vi "crh_xcopy.vi"() -> ()   [LabVIEW 2012]
panel:
  out "concatenated string":string
  out "OK 2":bool
  out "concatenated string 2":string
  out "folder 2":string
  out "OK":bool
  in  "folder":string="QAMT01\\CRH3605"
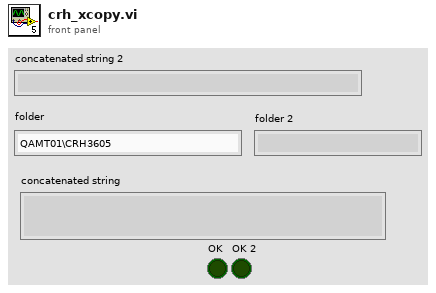
[diagram p1: front panel]
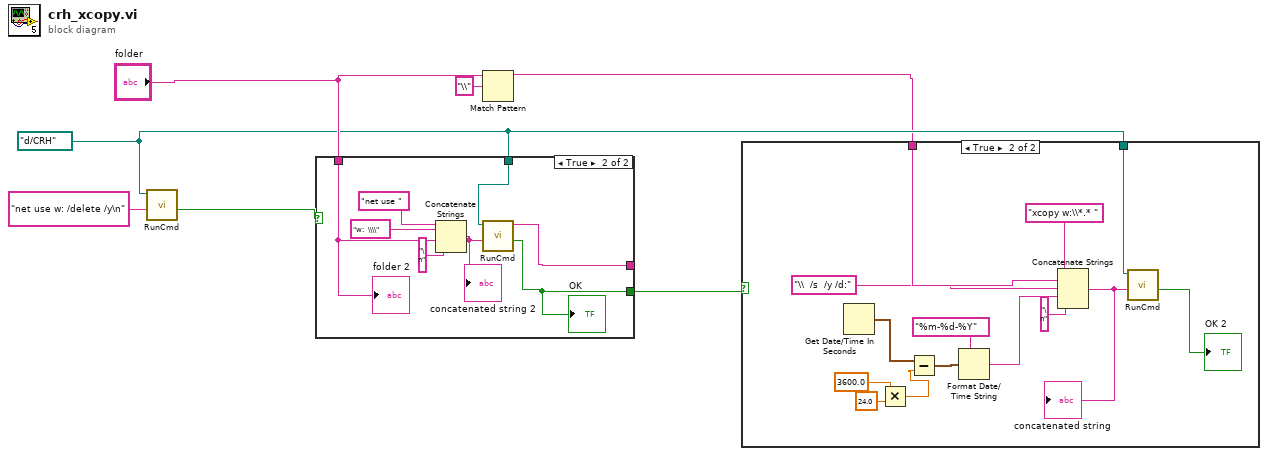
[diagram p0: block diagram]
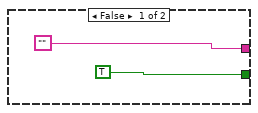
[diagram p3: hidden frame]
diagram:
  w3 = path "d:/CRH" ("working directory")
  n1 = call "RunCmd.vi"("Cmd String"="net use w: /delete /y\n" ("string"), "working directory"=w3) -> ("OK"=w1:bool)  [unwired: 8 in, 1 out]
  n2 = case shown="True" w1 {
    tunnel: [TRUE w11] -> w5
    tunnel: ["" w12] -> _
    tunnel: "folder" -> [_ w14]
    tunnel: w3 -> [_ w13]
    frame False {
    }
    frame True {
      n3 = Concatenate Strings("net use " ("string"), "w:  \\\\" ("string"), w14, "\n" ("string")) -> (w17:string)
      "concatenated string 2" <- w17
      n4 = call "RunCmd.vi"("Cmd String"=w17, "working directory"=w13) -> ("OK"=w11:bool, "Output"=w12:string)  [unwired: 8 in]
      "OK" <- w11
      "folder 2" <- w14
    }
  }
  n5 = Match Pattern(string="folder", regular expression="\\") -> (before substring=w2:string)  [unwired: 1 in, 3 out]
  n6 = case shown="True" w5 {
    tunnel: w2 -> [_ w31]
    tunnel: w3 -> [_ w22]
    frame False {
    }
    frame True {
      n7 = Get Date/Time In Seconds() -> (seconds since 1Jan1904=w24:timestamp)
      n8 = Multiply(x=3600.0, y=24.0) -> (x*y=w26:dbl)
      n9 = Subtract(x=w24, y=w26) -> (x-y=w27:timestamp)
      n10 = Format Date/Time String(time format string (%c)="%m-%d-%Y", seconds (now)=w27) -> (date/time string=w18:string)  [unwired: 1 in]
      n11 = Concatenate Strings("xcopy w:\\*.* " ("string"), w31, "\\  /s  /y /d:" ("string"), w18, "\n" ("string")) -> (w21:string)
      "concatenated string" <- w21
      n12 = call "RunCmd.vi"("Cmd String"=w21, "working directory"=w22) -> ("OK"=→"OK 2":bool)  [unwired: 8 in, 1 out]
    }
  }
